vi "trace_and_wait.vi"(8 "error in":errorcluster, 10 "Override":T1, 11 "Stimulus":T2 {"Length" min=0.0 max=100.0 step=100.0 format="%#_4p"; "Frequency" min=0.0 step=100.0 format="%#_4g"; "Offset" format="%#_3p"; "Amplitude" format="%#_3p"; "Phase" min=-180.0 max=360.0 step=100.0 format="%#.2f"}) -> (0 "error out":errorcluster)   [LabVIEW 2013]
uses:
  stimulus.ctl
  injection_point.ctl
  ui_override_opts.ctl
  initialization/micron_globals.vi
panel:
  # "This VI sets the stimulus, triggers a trace cycle, then waits for it to complete.  Use with ui_override.vi and single_trigger_setup.vi.  This is intended for programmatic sequencing of particular trace conditions."
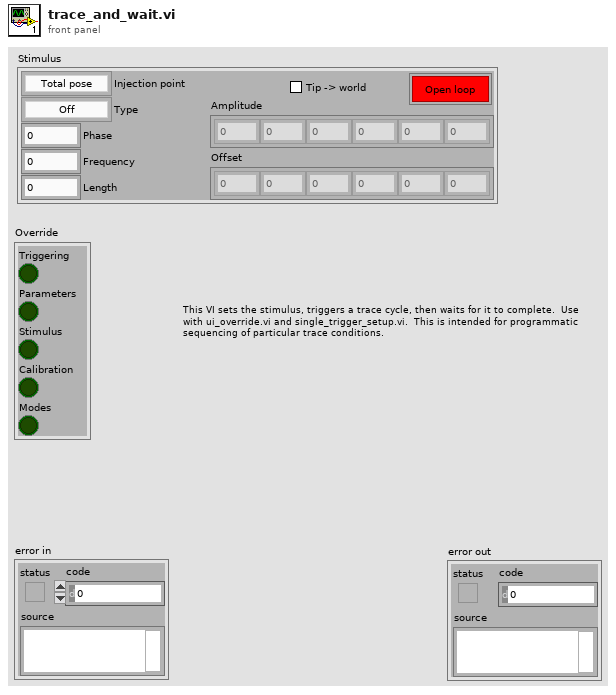
[diagram p1: front panel]
types:
  T1 = typedef "ui_override_opts.ctl" = cluster{"Triggering":bool, "Parameters":bool, "Stimulus":bool, "Calibration":bool, "Modes":bool}
  T2 = typedef "stimulus.ctl" = cluster{"Type":enum16{"Off", "Step", "Sine", "Triangle", "Arbitrary"}, "Phase":dbl, "Amplitude":sgl[], "Injection point":T3, "Closed loop":bool, "Offset":sgl[], "Tip -> world":bool, "Frequency":dbl, "Length":dbl}
  T3 = typedef "injection_point.ctl" = enum16{"Total pose", "V limiter", "Goal ", "Link position", "KF link position", "Inverse kin", "Link goal", "Link error", "Controller", "Output", "Drive", "Light"}
  T4 = typedef "micron_config.ctl" = cluster{"rt fifo":refnum<k33>, "Analog output task":refnum<k21>, "Analog output task 2":refnum<k21>, "Stimulus AO task":refnum<k21>, "Low-rate AIN task":refnum<k21>, "Pedal out task":refnum<k21>, "Pedal in task":refnum<k21>, "Loop timing source":string, "Relay out task":refnum<k21>, "Send UDP Conn":refnum<k16>, "Recv UDP Conn":refnum<k16>, "Host Addr":dbl, "I2C interface":T5, "trace_start notifier":refnum<notifier>, "trace_done notifier":refnum<notifier>, "ASAP FIFO":refnum<k33>}
  T5 = typedef "i2c_interface.ctl" = cluster{"FPGA VI Reference":T6}
  T6 = typedef "fpga_reference.ctl" = refnum<k20>
  T7 = typedef "Micron params.ctl" = cluster{"Stimulus":T2, "Goal Filter A":T8, "Mode controls":T9, "Manipulator type":enum16{"Current piezo", "Voltage piezo"}, "Manipulator calibration":T10, "Network":T12, "Goal Filter B":T8, "Cancellation":T13, "Transition time":sgl, "Estimation":T15}
  T8 = typedef "goal_loop_parms.ctl" = cluster{"Speedup max":sgl, "Speedup thresh":sgl, "Speedup nonlin":sgl, "Filters":cluster{"Lower Fc":sgl, "Lower Q":sgl, "Scale factor":sgl, "Upper Fc":sgl, "Upper Q":sgl, "V limit":sgl, "V limit range":sgl}[]}
  T9 = typedef "mode_conrols.ctl" = cluster{"Hold":bool, "Cancellation":bool, "Goal filter":bool, "Trigger":bool}
  T10 = typedef "manipulator_cal.ctl" = cluster{"Tool offsets":sgl[][], "Tip light calibration":T11, "Handle light calibration":T11, "Base pivots":sgl[][], "Output pivots":sgl[][], "Length center":sgl, "Workspace height":sgl[], "Workspace diameter":sgl[], "Linearization":sgl[][], "Stack travel":sgl, "Saturation pos":sgl, "Inverse filters":cluster{"filter structure":enum32{"IIR 2nd Order", "IIR 4th Order"}, "Reverse Coefficients":dbl[], "Forward Coefficients":dbl[]}[]}
  T11 = typedef "probe_calibration.ctl" = sgl[][]
  T12 = typedef "network_params.ctl" = cluster{"Remote Host":string, "Send Status":bool, "Send Port":u16, "Recv Commands":bool, "Recv Port":u16}
  T13 = typedef "sq_control_params.ctl" = cluster{"KP":T14, "KI":sgl, "KD":T14, "Max vel":sgl, "Max acc":sgl, "Int error limit":sgl, "RCM gain":sgl, "Bypass":bool, "Degraded gain":sgl}
  T14 = typedef "decoupled_gain.ctl" = cluster{"XY":sgl, "Rxy":sgl, "Z":sgl, "Rz":sgl}
  T15 = typedef "estimation_controls.ctl" = cluster{"Link":cluster{"Measure noise":dbl[], "Process noise":dbl[], "Alt process noise":dbl[], "Alt turnoff cycles":i32, "Innovation limit":dbl[], "Residue threshold":dbl, "Enable":bool}, "Handle":cluster{"Measure noise":dbl[], "Process noise":dbl[], "State limits":dbl[], "Innovation limit":dbl[], "Prediction Lookahead":sgl, "Enable":bool}}
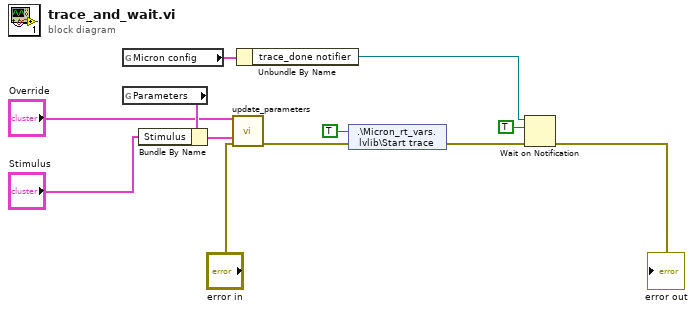
[diagram p0: block diagram]
diagram:
  n1 = global read "micron_globals.vi" "Micron config"() -> (w8:T4)
  n2 = global read "micron_globals.vi" "Parameters"() -> (w11:T7)
  n3 = Bundle By Name(cluster=w11, "Stimulus"="Stimulus") -> (w12:T7)
  n4 = call "update_parameters.vi"("Modify"="Override", "Parameters"=w12, "error in"="error in") -> ("error out"=w2:errorcluster)  [unwired: 11 in, 1 out]
  n5 = Unbundle By Name(w8) -> ("trace_done notifier"=w9:refnum<notifier>)
  n6 = shared-variable ".\\Micron_rt_vars.lvlib\\Start trace"(TRUE ("Start trace"), error in=w2) -> (error out=w1:errorcluster)
  n7 = Wait on Notification(notifier=w9, ignore previous (F)=TRUE, error in (no error)=w1) -> (error out=→"error out":errorcluster)  [unwired: 1 in, 3 out]
